vi "Car wash.vi"() -> ()   [LabVIEW 2015]
uses:
  USB Template (LV 8.6)/Car Wash/Controls/Car Wash Indicators.ctl
  USB Template (LV 8.6)/Car Wash/Controls/Wash Options.ctl
  status.ctl
  eash data.ctl
  times.ctl
  timerstatus.ctl
panel:
  in  "Wash Options":T1
  out "error out":errorcluster
  in  "error in":errorcluster
  in  "Start":bool
  out "Elapsed Time":dbl format="%0.2f"
  in  "stop":bool
  out "Wash Entry":bool
  in  "Car Position Slider":u8(slide) max=3 scale=0.0..4.0
  out "Car Wash Indicators":T2
  # "Entry Console"
  # "Car Wash Display"
  # "Car Position Simulation"
  # "Pre-Soak\nH-P Wash\nL-P Wax\nSpot Free Rinse"
  # "Underbody Wash\nBug Remover"
  # "Tire Shine\nAir Dry"
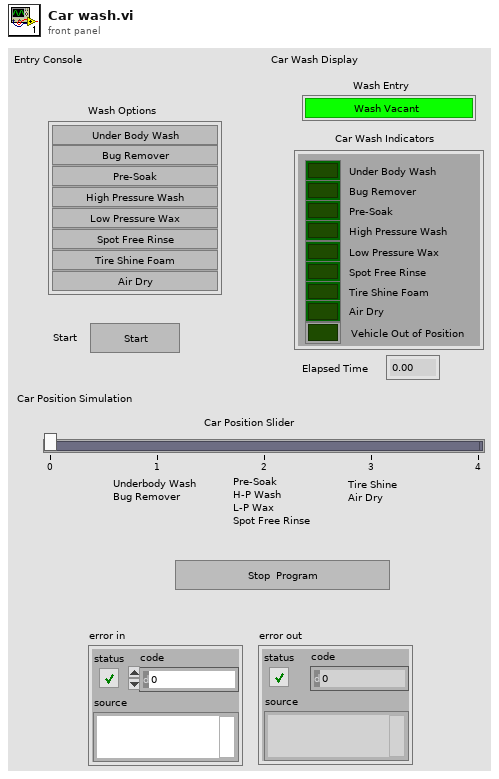
[diagram p1: front panel]
types:
  T1 = typedef "Wash Options.ctl" = cluster{"Underbody Wash":bool, "Bug Remover":bool, "Pre-Soak":bool, "High Pressure Wash":bool, "Low Pressure Wax":bool, "Spot Free Rinse":bool, "Tire Shine Foam":bool, "Air Dry":bool}
  T2 = typedef "Car Wash Indicators.ctl" = cluster{"Under Body Wash":bool, "Bug Remover":bool, "Pre-Soak":bool, "High Pressure Wash":bool, "Low Pressure Wax":bool, "Spot Free Rinse":bool, "Tire Shine Foam":bool, "Air Dry":bool, "Vehicle Out of Position":bool}
  T3 = typedef "status.ctl" = enum16{"AD", "End", "TSF", "SFR", "LPW", "HPW", "P-S", "BR", "UBW", "Exit", "Error", "Idle", "Initialize"}
  T4 = enum8{"Enabled", "Disabled", "Disabled and Grayed Out"}
  T5 = typedef "timerstatus.ctl" = enum16{"Pause", "Stop", "Start"}
  T6 = typedef "eash data.ctl" = cluster{"Wash Options":T1, "times":T7, "Car Wash Indicators":T2, "wash entry":bool, "time ":dbl}
  T7 = typedef "times.ctl" = cluster{"UBW":dbl, "BR":dbl, "P-S":dbl, "HPW":dbl, "LPW":dbl, "SFR":dbl, "AD":dbl}
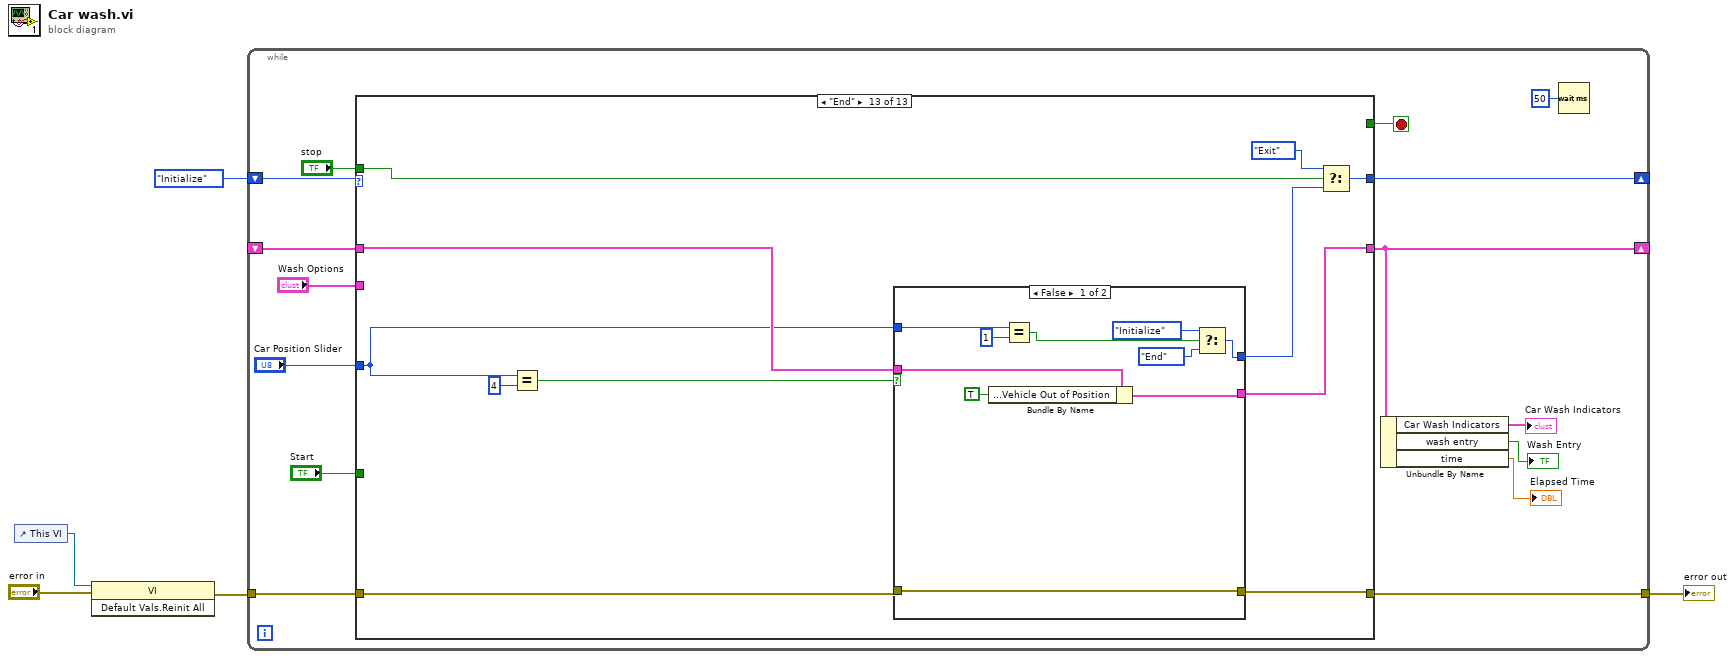
[diagram p0: block diagram]
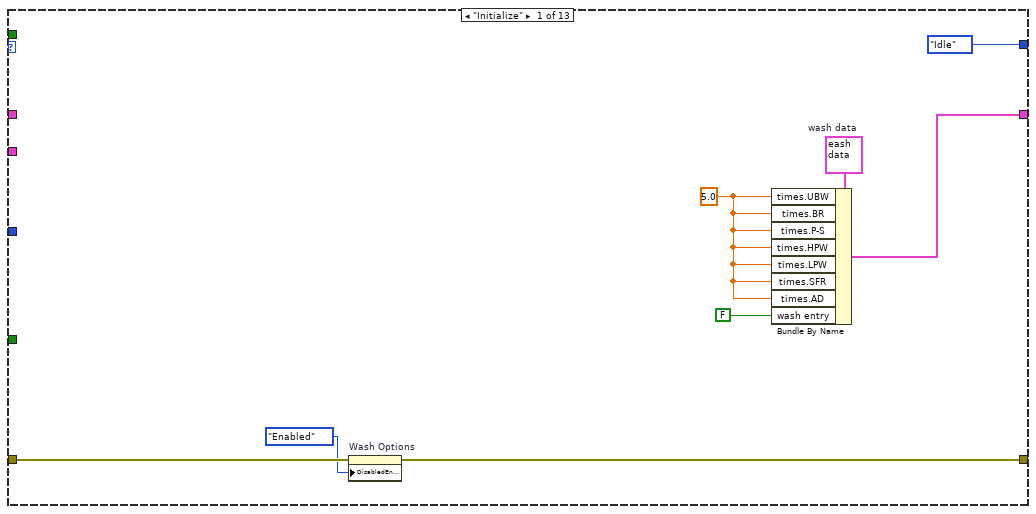
[diagram p2: hidden frame]
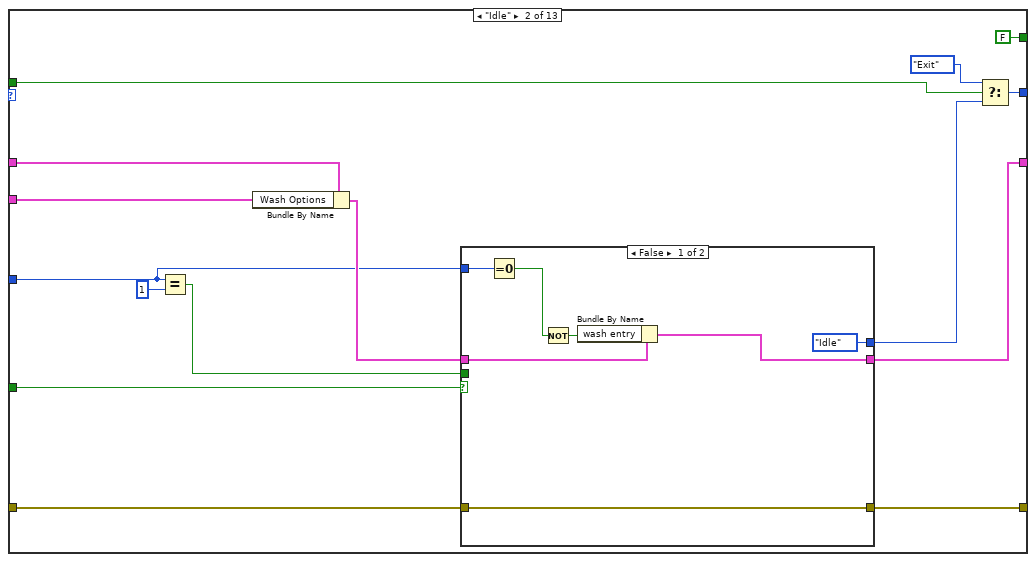
[diagram p3: hidden frame]
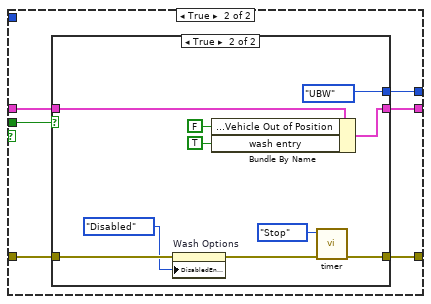
[diagram p4: hidden frame]
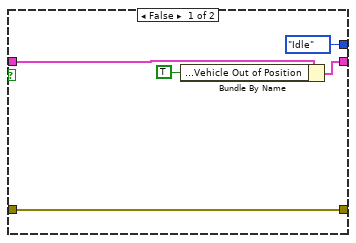
[diagram p5: hidden frame]
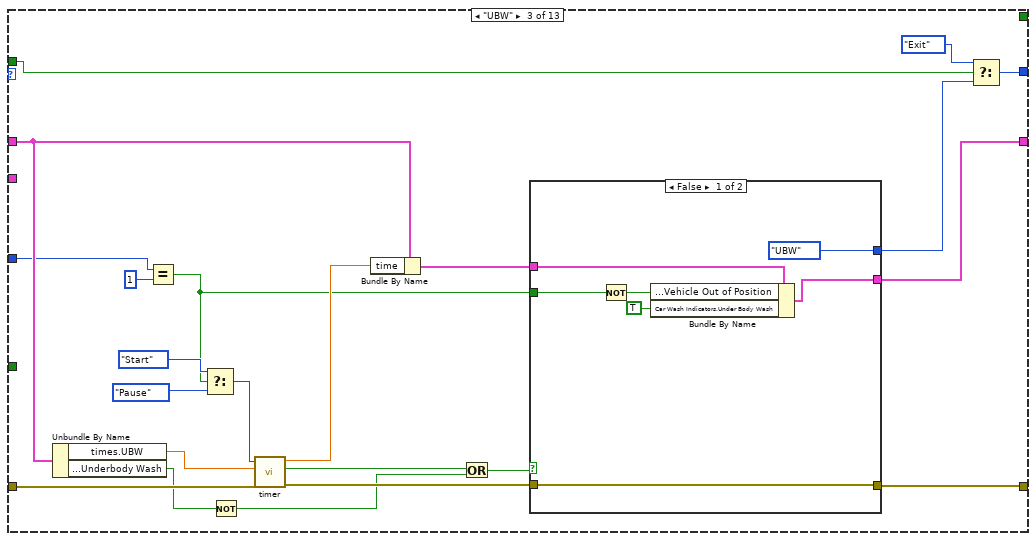
[diagram p6: hidden frame]
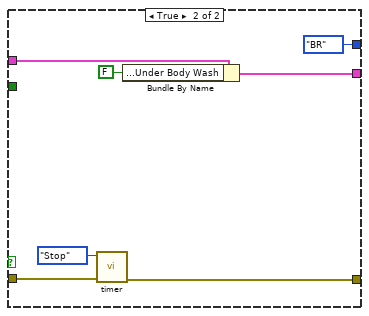
[diagram p7: hidden frame]
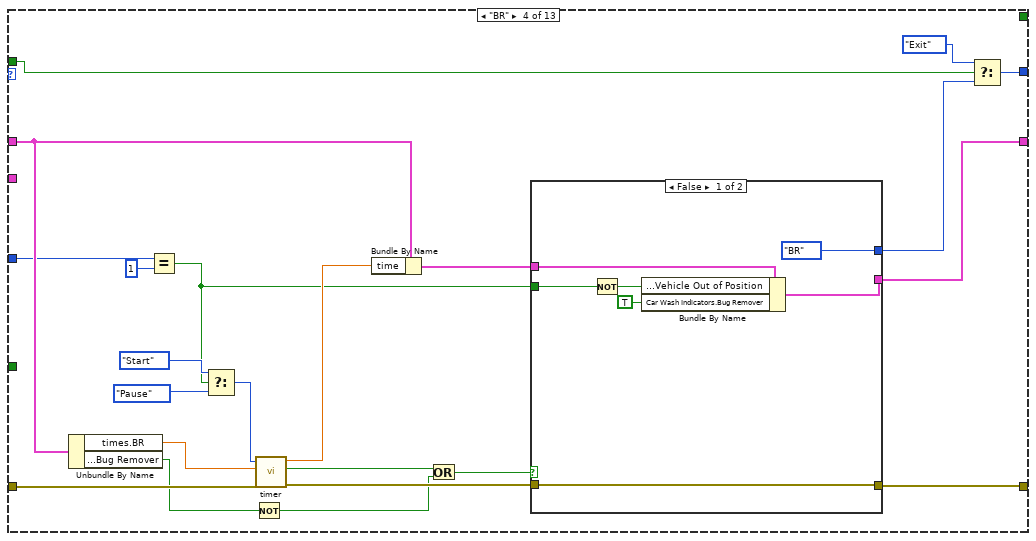
[diagram p8: hidden frame]
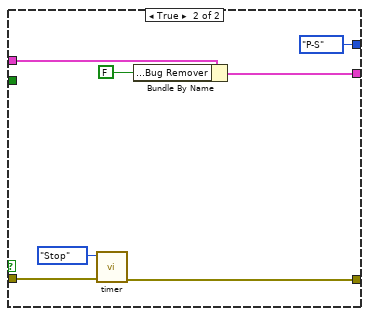
[diagram p9: hidden frame]
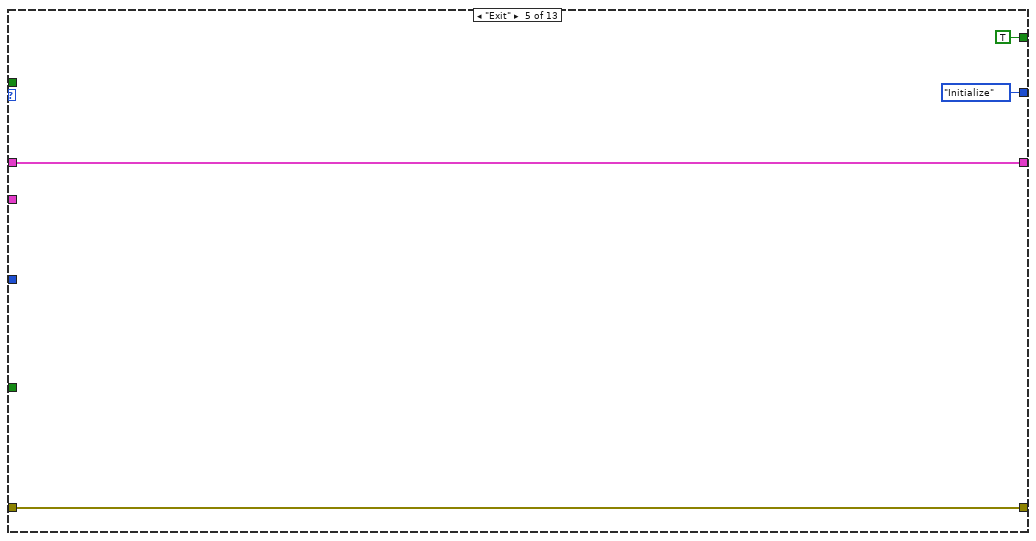
[diagram p10: hidden frame]
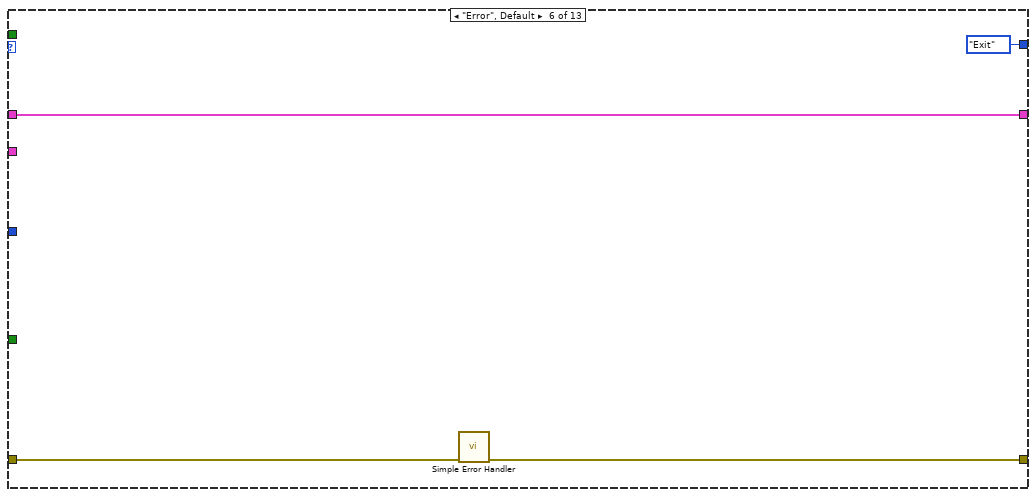
[diagram p11: hidden frame]
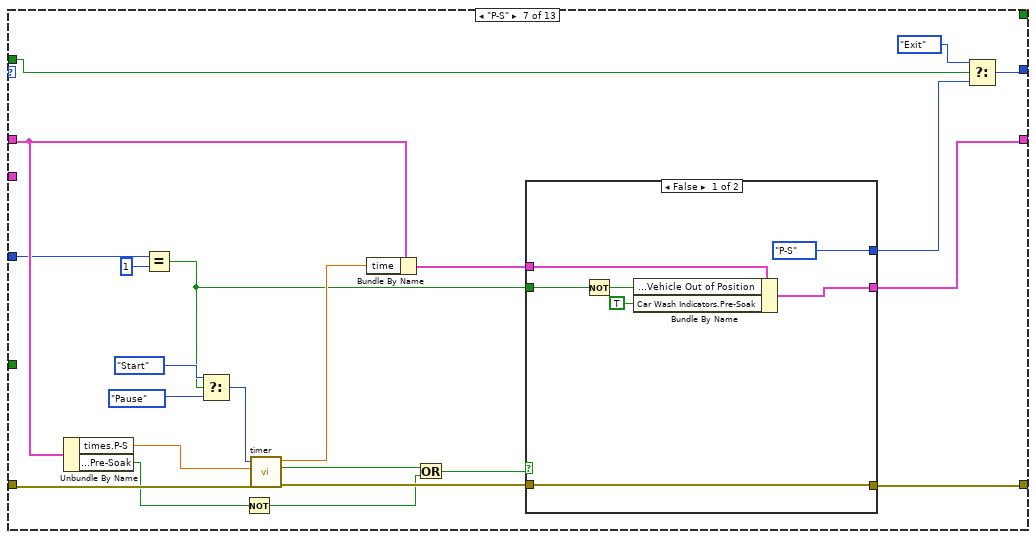
[diagram p12: hidden frame]
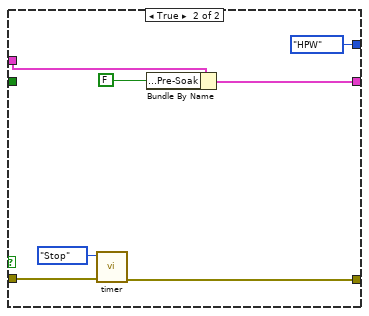
[diagram p13: hidden frame]
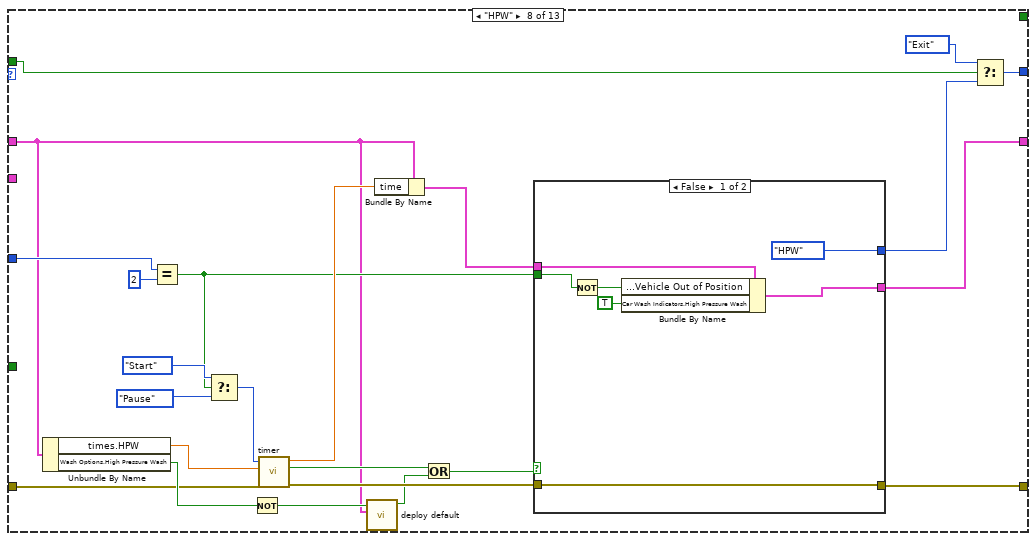
[diagram p14: hidden frame]
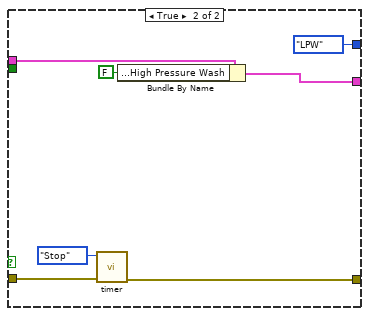
[diagram p15: hidden frame]
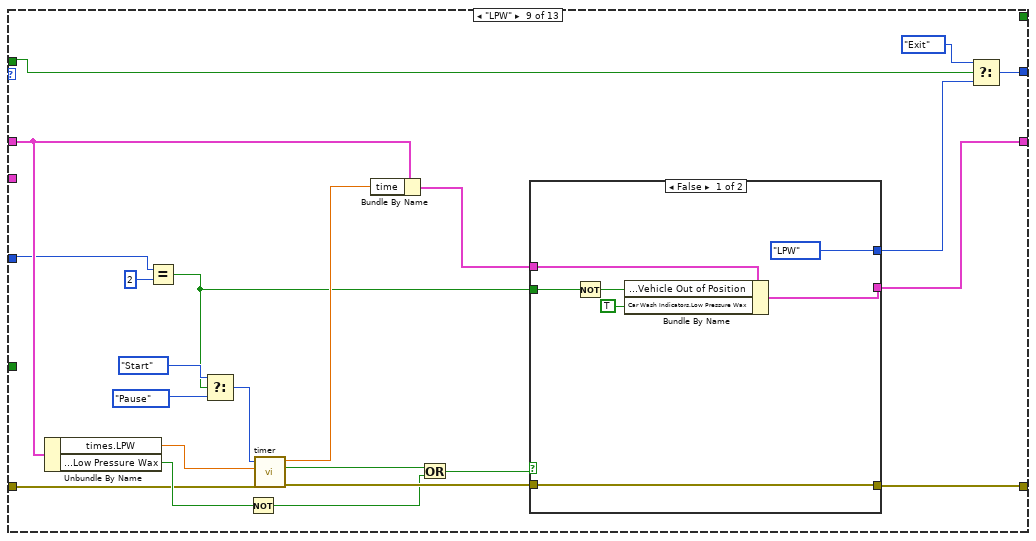
[diagram p16: hidden frame]
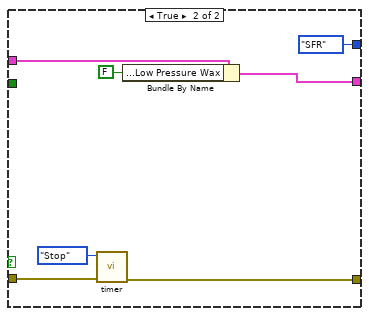
[diagram p17: hidden frame]
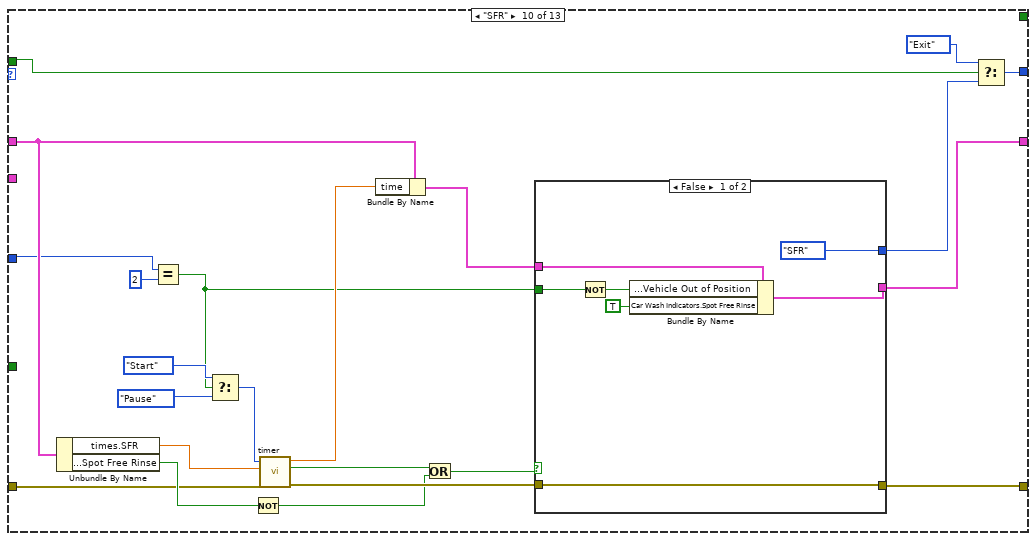
[diagram p18: hidden frame]
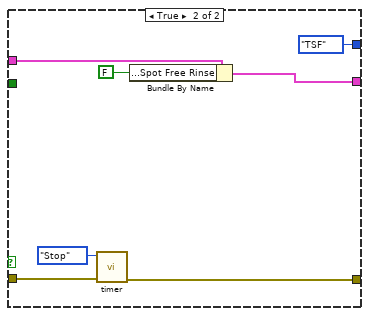
[diagram p19: hidden frame]
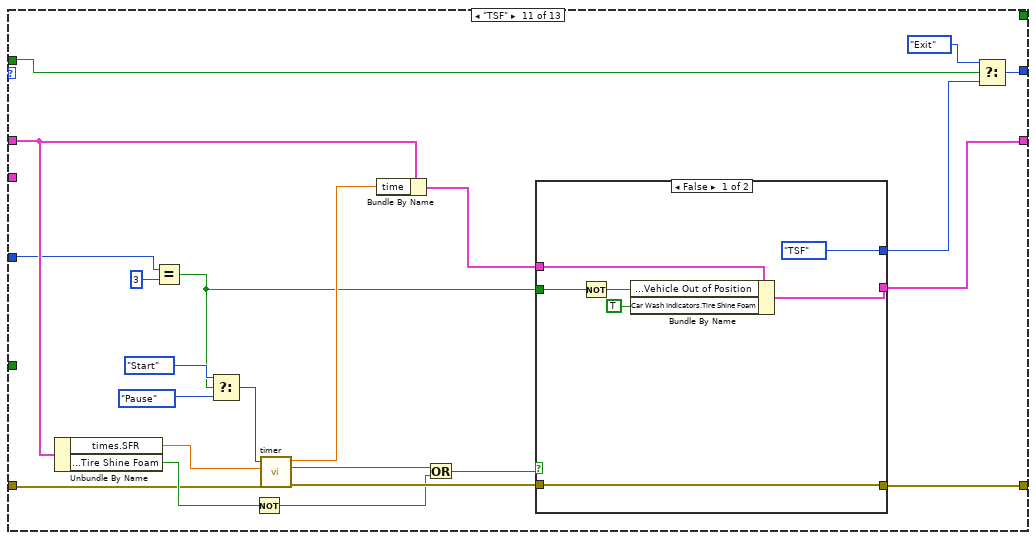
[diagram p20: hidden frame]
diagram:
  n1 = control-ref of="This VI"() -> (w3:refnum<vi>)
  n2 = invoke class="VI" method="Default Vals.Reinit All"(reference=w3, error in="error in") -> (error out=w2:errorcluster)  [unwired: 1 in, 2 out]
  n3 = while {
    tunnel: w2 -> [w20]
    tunnel: [w19] -> w5
    shift-right: [w10] -> _
    shift-left: _ -> [w16]
    shift-right: [w15] -> _
    shift-left: status."Initialize" ("status") -> [w17]
    stop <- w18 stop-if-true
    n4 = case shown="\"End\"" w17 {
      tunnel: w20 -> [w24 w41 w93 w120 w146 w150 w164 w200 w233 w268 w304 w340 w374]
      tunnel: [w23 w38 w79 w119 w146 w148 w163 w199 w232 w267 w303 w339 w377] -> w19
      tunnel: [_ FALSE _ _ TRUE _ _ _ _ _ _ _ _] -> w18
      tunnel: [w26 w37 w80 w116 w147 w151 w161 w198 w229 w265 w302 w337 w376] -> w10
      tunnel: w16 -> [_ w43 w91 w118 w147 w151 w162 w189 w230 w266 w301 w338 w372]
      tunnel: [status."Idle" ("status") w33 w89 w115 status."Initialize" ("t") status."Exit" ("t") w159 w195 w228 w264 w299 w336 w371] -> w15
      tunnel: "Wash Options" -> [_ w42 _ _ _ _ _ _ _ _ _ _ _]
      tunnel: "Car Position Slider" -> [_ w30 w73 w109 _ _ w153 w194 w226 w262 w298 w334 w369]
      tunnel: "Start" -> [_ w29 _ _ _ _ _ _ _ _ _ _ _]
      tunnel: "stop" -> [_ w34 w88 w117 _ _ w160 w197 w231 w263 w300 w335 w375]
      frame "Initialize" {
        w28 = T6 {"Wash Options"={"Underbody Wash"=FALSE, "Bug Remover"=FALSE, "Pre-Soak"=FALSE, "High Pressure Wash"=FALSE, "Low Pressure Wax"=FALSE, "Spot Free Rinse"=FALSE, "Tire Shine Foam"=FALSE, "Air Dry"=FALSE}, "times"={"UBW"=0.0, "BR"=0.0, "P-S"=0.0, "HPW"=0.0, "LPW"=0.0, "SFR"=0.0, "AD"=0.0}, "Car Wash Indicators"={"Under Body Wash"=FALSE, "Bug Remover"=FALSE, "Pre-Soak"=FALSE, "High Pressure Wash"=FALSE, "Low Pressure Wax"=FALSE, "Spot Free Rinse"=FALSE, "Tire Shine Foam"=FALSE, "Air Dry"=FALSE, "Vehicle Out of Position"=FALSE}, "wash entry"=FALSE, "time "=0.0}  # wash data
        w27 = 5.0 ("times.UBW")
        n5 = property on="Wash Options" class="Clust (strict)"(error in=w24, "DisabledEnum"=T4."Enabled" ("Disabled")) -> (error out=w23:errorcluster)  [unwired: 1 in, 1 out]
        n6 = Bundle By Name(cluster=w28, "times.UBW"=w27, "times.BR"=w27, "times.P-S"=w27, "times.HPW"=w27, "times.LPW"=w27, "times.SFR"=w27, "times.AD"=w27, "wash entry"=FALSE ("Car Wash Indicators.Vehicle Out of Position")) -> (w26:T6)
      }
      frame "Idle" {
        n7 = Equal?(x=w30, y=u8 1) -> (x = y?=w40:bool)
        n8 = Bundle By Name(cluster=w43, "Wash Options"=w42) -> (w39:T6)
        n9 = case shown="False" w29 {
          tunnel: w41 -> [w49 w56]
          tunnel: w40 -> [_ w54]
          tunnel: w39 -> [w47 w53]
          tunnel: [w49 w55] -> w38
          tunnel: [status."Idle" ("status") w52] -> w35
          tunnel: [w46 w51] -> w37
          tunnel: w30 -> [w48 _]
          frame False {
            n10 = Equal To 0?(x=w48) -> (x = 0?=w44:bool)
            n11 = Not(x=w44) -> (.not. x?=w45:bool)
            n12 = Bundle By Name(cluster=w47, "wash entry"=w45) -> (w46:T6)
          }
          frame True {
            n13 = case shown="True" w54 {
              tunnel: w56 -> [w57 w65]
              tunnel: [w57 w67] -> w55
              tunnel: w53 -> [w60 w70]
              tunnel: [status."Idle" ("status") status."UBW" ("status")] -> w52
              tunnel: [w58 w69] -> w51
              frame False {
                n14 = Bundle By Name(cluster=w60, "Car Wash Indicators.Vehicle Out of Position"=TRUE ("Car Wash Indicators 2.Vehicle Out of Position")) -> (w58:T6)
              }
              frame True {
                n15 = property on="Wash Options" class="Clust (strict)"(error in=w65, "DisabledEnum"=T4."Disabled" ("Disabled")) -> (error out=w64:errorcluster)  [unwired: 1 in, 1 out]
                n16 = Bundle By Name(cluster=w70, "Car Wash Indicators.Vehicle Out of Position"=FALSE ("Car Wash Indicators 2.Vehicle Out of Position"), "wash entry"=TRUE) -> (w69:T6)
                n17 = call "timer.vi"("error in"=w64, "timerstatus"=timerstatus."Stop") -> ("error out"=w67:errorcluster)  [unwired: 7 in, 2 out]
              }
            }
          }
        }
        n18 = Select(t=status."Exit", s=w34, f=w35) -> (s? t:f=w33:T3)
      }
      frame "UBW" {
        n19 = Unbundle By Name(w91) -> ("times.UBW"=w92:dbl, "Wash Options.Underbody Wash"=w77:bool)
        n20 = Equal?(x=w73, y=u8 1) -> (x = y?=w74:bool)
        n21 = Select(t=timerstatus."Start" ("timerstatus"), s=w74, f=timerstatus."Pause" ("timerstatus")) -> (s? t:f=w82:T5)
        n22 = Not(x=w77) -> (.not. x?=w75:bool)
        n23 = call "timer.vi"("error in"=w93, "limit"=w92, "timerstatus"=w82) -> ("error out"=w87:errorcluster, "limit out"=w78:bool, "elapsed"=w86:dbl)  [unwired: 6 in]
        n24 = Bundle By Name(cluster=w91, "time"=w86) -> (w85:T6)
        n25 = Or(x=w78, y=w75) -> (x .or. y?=w76:bool)
        n26 = case shown="False" w76 {
          tunnel: w87 -> [w99 w107]
          tunnel: w85 -> [w97 w103]
          tunnel: [status."UBW" ("t") status."BR" ("t")] -> w81
          tunnel: [w96 w102] -> w80
          tunnel: [w99 w106] -> w79
          tunnel: w74 -> [w95 _]
          frame False {
            n27 = Not(x=w95) -> (.not. x?=w98:bool)
            n28 = Bundle By Name(cluster=w97, "Car Wash Indicators.Vehicle Out of Position"=w98, "Car Wash Indicators.Under Body Wash"=TRUE) -> (w96:T6)
          }
          frame True {
            n29 = call "timer.vi"("error in"=w107, "timerstatus"=timerstatus."Stop") -> ("error out"=w106:errorcluster)  [unwired: 7 in, 2 out]
            n30 = Bundle By Name(cluster=w103, "Car Wash Indicators.Under Body Wash"=FALSE) -> (w102:T6)
          }
        }
        n31 = Select(t=status."Exit", s=w88, f=w81) -> (s? t:f=w89:T3)
      }
      frame "BR" {
        n32 = Unbundle By Name(w118) -> ("times.BR"=w121:dbl, "Wash Options.Bug Remover"=w114:bool)
        n33 = Equal?(x=w109, y=u8 1) -> (x = y?=w110:bool)
        n34 = Select(t=timerstatus."Start" ("timerstatus"), s=w110, f=timerstatus."Pause" ("timerstatus")) -> (s? t:f=w128:T5)
        n35 = Not(x=w114) -> (.not. x?=w113:bool)
        n36 = call "timer.vi"("error in"=w120, "limit"=w121, "timerstatus"=w128) -> ("error out"=w123:errorcluster, "limit out"=w112:bool, "elapsed"=w124:dbl)  [unwired: 6 in]
        n37 = Bundle By Name(cluster=w118, "time"=w124) -> (w125:T6)
        n38 = Or(x=w112, y=w113) -> (x .or. y?=w111:bool)
        n39 = case shown="False" w111 {
          tunnel: w123 -> [w135 w143]
          tunnel: w125 -> [w133 w139]
          tunnel: [status."BR" ("t") status."P-S" ("t")] -> w129
          tunnel: [w132 w138] -> w116
          tunnel: [w135 w142] -> w119
          tunnel: w110 -> [w131 _]
          frame False {
            n40 = Not(x=w131) -> (.not. x?=w134:bool)
            n41 = Bundle By Name(cluster=w133, "Car Wash Indicators.Vehicle Out of Position"=w134, "Car Wash Indicators.Bug Remover"=TRUE ("Wash Options.Bug Remover")) -> (w132:T6)
          }
          frame True {
            n42 = call "timer.vi"("error in"=w143, "timerstatus"=timerstatus."Stop") -> ("error out"=w142:errorcluster)  [unwired: 7 in, 2 out]
            n43 = Bundle By Name(cluster=w139, "Car Wash Indicators.Bug Remover"=FALSE ("Car Wash Indicators.Under Body Wash")) -> (w138:T6)
          }
        }
        n44 = Select(t=status."Exit", s=w117, f=w129) -> (s? t:f=w115:T3)
      }
      frame "Exit" {
      }
      frame "Error", Default {
        n45 = call <vilib>:"Simple Error Handler.vi"("error in (no error)"=w150) -> ("error out"=w148:errorcluster)  [unwired: 4 in, 4 out]
      }
      frame "P-S" {
        n46 = Unbundle By Name(w162) -> ("times.P-S"=w173:dbl, "Wash Options.Pre-Soak"=w158:bool)
        n47 = Equal?(x=w153, y=u8 1) -> (x = y?=w154:bool)
        n48 = Select(t=timerstatus."Start" ("timerstatus"), s=w154, f=timerstatus."Pause" ("timerstatus")) -> (s? t:f=w166:T5)
        n49 = Not(x=w158) -> (.not. x?=w157:bool)
        n50 = call "timer.vi"("error in"=w164, "limit"=w173, "timerstatus"=w166) -> ("error out"=w171:errorcluster, "limit out"=w156:bool, "elapsed"=w170:dbl)  [unwired: 6 in]
        n51 = Bundle By Name(cluster=w162, "time"=w170) -> (w169:T6)
        n52 = Or(x=w156, y=w157) -> (x .or. y?=w155:bool)
        n53 = case shown="False" w155 {
          tunnel: w171 -> [w179 w187]
          tunnel: w169 -> [w177 w183]
          tunnel: [status."P-S" ("t") status."HPW" ("t")] -> w165
          tunnel: [w176 w182] -> w161
          tunnel: [w179 w186] -> w163
          tunnel: w154 -> [w175 _]
          frame False {
            n54 = Not(x=w175) -> (.not. x?=w178:bool)
            n55 = Bundle By Name(cluster=w177, "Car Wash Indicators.Vehicle Out of Position"=w178, "Car Wash Indicators.Pre-Soak"=TRUE) -> (w176:T6)
          }
          frame True {
            n56 = call "timer.vi"("error in"=w187, "timerstatus"=timerstatus."Stop") -> ("error out"=w186:errorcluster)  [unwired: 7 in, 2 out]
            n57 = Bundle By Name(cluster=w183, "Car Wash Indicators.Pre-Soak"=FALSE ("Car Wash Indicators.Under Body Wash")) -> (w182:T6)
          }
        }
        n58 = Select(t=status."Exit", s=w160, f=w165) -> (s? t:f=w159:T3)
      }
      frame "HPW" {
        n59 = Unbundle By Name(w189) -> ("times.HPW"=w210:dbl, "Wash Options.High Pressure Wash"=w202:bool)
        n60 = Equal?(x=w194, y=u8 2) -> (x = y?=w196:bool)
        n61 = Select(t=timerstatus."Start" ("timerstatus"), s=w196, f=timerstatus."Pause" ("timerstatus")) -> (s? t:f=w204:T5)
        n62 = Not(x=w202) -> (.not. x?=w191:bool)
        n63 = call "timer.vi"("error in"=w200, "limit"=w210, "timerstatus"=w204) -> ("error out"=w208:errorcluster, "limit out"=w201:bool, "elapsed"=w207:dbl)  [unwired: 6 in]
        n64 = call "deploy default.vi"("data"=w189, "in"=w191) -> ("deploy"=w190:bool)  [unwired: 9 in]
        n65 = Bundle By Name(cluster=w189, "time"=w207) -> (w192:T6)
        n66 = Or(x=w201, y=w190) -> (x .or. y?=w188:bool)
        n67 = case shown="False" w188 {
          tunnel: w208 -> [w216 w224]
          tunnel: w192 -> [w213 w220]
          tunnel: [status."HPW" ("t") status."LPW" ("t")] -> w203
          tunnel: [w212 w219] -> w198
          tunnel: [w216 w223] -> w199
          tunnel: w196 -> [w214 _]
          frame False {
            n68 = Not(x=w214) -> (.not. x?=w215:bool)
            n69 = Bundle By Name(cluster=w213, "Car Wash Indicators.Vehicle Out of Position"=w215, "Car Wash Indicators.High Pressure Wash"=TRUE) -> (w212:T6)
          }
          frame True {
            n70 = call "timer.vi"("error in"=w224, "timerstatus"=timerstatus."Stop") -> ("error out"=w223:errorcluster)  [unwired: 7 in, 2 out]
            n71 = Bundle By Name(cluster=w220, "Car Wash Indicators.High Pressure Wash"=FALSE ("Car Wash Indicators.Under Body Wash")) -> (w219:T6)
          }
        }
        n72 = Select(t=status."Exit", s=w197, f=w203) -> (s? t:f=w195:T3)
      }
      frame "LPW" {
        n73 = Unbundle By Name(w230) -> ("times.LPW"=w246:dbl, "Wash Options.Low Pressure Wax"=w237:bool)
        n74 = Equal?(x=w226, y=u8 2) -> (x = y?=w227:bool)
        n75 = Select(t=timerstatus."Start" ("timerstatus"), s=w227, f=timerstatus."Pause" ("timerstatus")) -> (s? t:f=w239:T5)
        n76 = Not(x=w237) -> (.not. x?=w236:bool)
        n77 = call "timer.vi"("error in"=w233, "limit"=w246, "timerstatus"=w239) -> ("error out"=w244:errorcluster, "limit out"=w235:bool, "elapsed"=w243:dbl)  [unwired: 6 in]
        n78 = Bundle By Name(cluster=w230, "time"=w243) -> (w242:T6)
        n79 = Or(x=w235, y=w236) -> (x .or. y?=w234:bool)
        n80 = case shown="False" w234 {
          tunnel: w244 -> [w252 w260]
          tunnel: w242 -> [w251 w256]
          tunnel: [status."LPW" ("t") status."SFR" ("t")] -> w238
          tunnel: [w250 w255] -> w229
          tunnel: [w252 w259] -> w232
          tunnel: w227 -> [w248 _]
          frame False {
            n81 = Not(x=w248) -> (.not. x?=w249:bool)
            n82 = Bundle By Name(cluster=w251, "Car Wash Indicators.Vehicle Out of Position"=w249, "Car Wash Indicators.Low Pressure Wax"=TRUE ("wash entry")) -> (w250:T6)
          }
          frame True {
            n83 = call "timer.vi"("error in"=w260, "timerstatus"=timerstatus."Stop") -> ("error out"=w259:errorcluster)  [unwired: 7 in, 2 out]
            n84 = Bundle By Name(cluster=w256, "Car Wash Indicators.Low Pressure Wax"=FALSE ("Car Wash Indicators.Under Body Wash")) -> (w255:T6)
          }
        }
        n85 = Select(t=status."Exit", s=w231, f=w238) -> (s? t:f=w228:T3)
      }
      frame "SFR" {
        n86 = Unbundle By Name(w266) -> ("times.SFR"=w282:dbl, "Wash Options.Spot Free Rinse"=w273:bool)
        n87 = Equal?(x=w262, y=u8 2) -> (x = y?=w269:bool)
        n88 = Select(t=timerstatus."Start" ("timerstatus"), s=w269, f=timerstatus."Pause" ("timerstatus")) -> (s? t:f=w275:T5)
        n89 = Not(x=w273) -> (.not. x?=w272:bool)
        n90 = call "timer.vi"("error in"=w268, "limit"=w282, "timerstatus"=w275) -> ("error out"=w280:errorcluster, "limit out"=w271:bool, "elapsed"=w279:dbl)  [unwired: 6 in]
        n91 = Bundle By Name(cluster=w266, "time"=w279) -> (w278:T6)
        n92 = Or(x=w271, y=w272) -> (x .or. y?=w270:bool)
        n93 = case shown="False" w270 {
          tunnel: w280 -> [w288 w296]
          tunnel: w278 -> [w287 w292]
          tunnel: [status."SFR" ("t") status."TSF" ("t")] -> w274
          tunnel: [w286 w291] -> w265
          tunnel: [w288 w295] -> w267
          tunnel: w269 -> [w284 _]
          frame False {
            n94 = Not(x=w284) -> (.not. x?=w285:bool)
            n95 = Bundle By Name(cluster=w287, "Car Wash Indicators.Vehicle Out of Position"=w285, "Car Wash Indicators.Spot Free Rinse"=TRUE) -> (w286:T6)
          }
          frame True {
            n96 = call "timer.vi"("error in"=w296, "timerstatus"=timerstatus."Stop") -> ("error out"=w295:errorcluster)  [unwired: 7 in, 2 out]
            n97 = Bundle By Name(cluster=w292, "Car Wash Indicators.Spot Free Rinse"=FALSE ("Car Wash Indicators.Under Body Wash")) -> (w291:T6)
          }
        }
        n98 = Select(t=status."Exit", s=w263, f=w274) -> (s? t:f=w264:T3)
      }
      frame "TSF" {
        n99 = Unbundle By Name(w301) -> ("times.SFR"=w318:dbl, "Wash Options.Tire Shine Foam"=w309:bool)
        n100 = Equal?(x=w298, y=u8 3) -> (x = y?=w305:bool)
        n101 = Select(t=timerstatus."Start" ("timerstatus"), s=w305, f=timerstatus."Pause" ("timerstatus")) -> (s? t:f=w311:T5)
        n102 = Not(x=w309) -> (.not. x?=w308:bool)
        n103 = call "timer.vi"("error in"=w304, "limit"=w318, "timerstatus"=w311) -> ("error out"=w316:errorcluster, "limit out"=w307:bool, "elapsed"=w315:dbl)  [unwired: 6 in]
        n104 = Bundle By Name(cluster=w301, "time"=w315) -> (w314:T6)
        n105 = Or(x=w307, y=w308) -> (x .or. y?=w306:bool)
        n106 = case shown="False" w306 {
          tunnel: w316 -> [w324 w332]
          tunnel: w314 -> [w323 w328]
          tunnel: [status."TSF" ("t") status."AD" ("t")] -> w310
          tunnel: [w322 w327] -> w302
          tunnel: [w324 w331] -> w303
          tunnel: w305 -> [w320 _]
          frame False {
            n107 = Not(x=w320) -> (.not. x?=w321:bool)
            n108 = Bundle By Name(cluster=w323, "Car Wash Indicators.Vehicle Out of Position"=w321, "Car Wash Indicators.Tire Shine Foam"=TRUE) -> (w322:T6)
          }
          frame True {
            n109 = call "timer.vi"("error in"=w332, "timerstatus"=timerstatus."Stop") -> ("error out"=w331:errorcluster)  [unwired: 7 in, 2 out]
            n110 = Bundle By Name(cluster=w328, "Car Wash Indicators.Tire Shine Foam"=FALSE ("Car Wash Indicators.Under Body Wash")) -> (w327:T6)
          }
        }
        n111 = Select(t=status."Exit", s=w300, f=w310) -> (s? t:f=w299:T3)
      }
      frame "AD" {
        n112 = Unbundle By Name(w338) -> ("times.AD"=w341:dbl, "Wash Options.Air Dry"=w350:bool)
        n113 = Equal?(x=w334, y=u8 3) -> (x = y?=w354:bool)
        n114 = Select(t=timerstatus."Start" ("timerstatus"), s=w354, f=timerstatus."Pause" ("timerstatus")) -> (s? t:f=w348:T5)
        n115 = Not(x=w350) -> (.not. x?=w351:bool)
        n116 = call "timer.vi"("error in"=w340, "limit"=w341, "timerstatus"=w348) -> ("error out"=w343:errorcluster, "limit out"=w352:bool, "elapsed"=w344:dbl)  [unwired: 6 in]
        n117 = Bundle By Name(cluster=w338, "time"=w344) -> (w345:T6)
        n118 = Or(x=w352, y=w351) -> (x .or. y?=w353:bool)
        n119 = case shown="True" w353 {
          tunnel: w343 -> [w360 w368]
          tunnel: w345 -> [w359 w364]
          tunnel: [status."LPW" ("t") status."End" ("t")] -> w349
          tunnel: [w358 w363] -> w337
          tunnel: [w360 w367] -> w339
          tunnel: w354 -> [w356 _]
          frame False {
            n120 = Not(x=w356) -> (.not. x?=w357:bool)
            n121 = Bundle By Name(cluster=w359, "Car Wash Indicators.Vehicle Out of Position"=w357, "Car Wash Indicators.Air Dry"=TRUE ("wash entry")) -> (w358:T6)
          }
          frame True {
            n122 = call "timer.vi"("error in"=w368, "timerstatus"=timerstatus."Stop") -> ("error out"=w367:errorcluster)  [unwired: 7 in, 2 out]
            n123 = Bundle By Name(cluster=w364, "Car Wash Indicators.Air Dry"=FALSE ("Car Wash Indicators.Under Body Wash")) -> (w363:T6)
          }
        }
        n124 = Select(t=status."Exit", s=w335, f=w349) -> (s? t:f=w336:T3)
      }
      frame "End" {
        n125 = Equal?(x=w369, y=u8 4) -> (x = y?=w373:bool)
        n126 = case shown="False" w373 {
          tunnel: w374 -> [w389 w391]
          tunnel: w372 -> [w388 w394]
          tunnel: [w380 status."End" ("t")] -> w378
          tunnel: [w387 w393] -> w376
          tunnel: [w389 w391] -> w377
          tunnel: w369 -> [w385 _]
          frame False {
            n127 = Bundle By Name(cluster=w388, "Car Wash Indicators.Vehicle Out of Position"=TRUE) -> (w387:T6)
            n128 = Equal?(x=w385, y=u8 1) -> (x = y?=w383:bool)
            n129 = Select(t=status."Initialize", s=w383, f=status."End" ("t")) -> (s? t:f=w380:T3)
          }
          frame True {
            n130 = Bundle By Name(cluster=w394, "Car Wash Indicators.Vehicle Out of Position"=FALSE ("Car Wash Indicators.Under Body Wash"), "wash entry"=FALSE) -> (w393:T6)
          }
        }
        n131 = Select(t=status."Exit", s=w375, f=w378) -> (s? t:f=w371:T3)
      }
    }
    n132 = Unbundle By Name(w10) -> ("Car Wash Indicators"=→"Car Wash Indicators":T2, "wash entry"=→"Wash Entry":bool, "time"=→"Elapsed Time":dbl)
    n133 = Wait (ms)(milliseconds to wait=u32 50) -> ()  [unwired: 1 out]
  }
  "error out" <- w5
